vi "Inline CRC-8-CCITT & CRC-8-Maxim.vi"(0 "CRC In":u8 format="%.0x", 1 "CRC-8 Type":T1(ring), 5 "Reset":bool, 7 "Data":u8 format="%.0x", 11 "error in (no error)":errorcluster) -> (4 "CRC":u8 format="%.0x", 15 "error out":errorcluster)   [LabVIEW 2020]
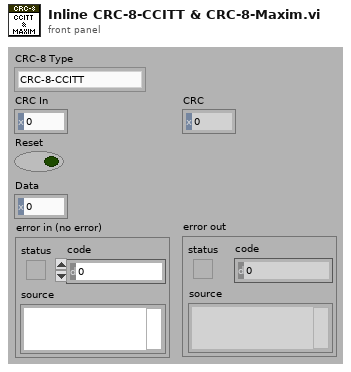
[diagram p1: front panel]
types:
  T1 = enum16{"CRC-8-CCITT", "CRC-8-Maxim 1-Wire (DOW)"}
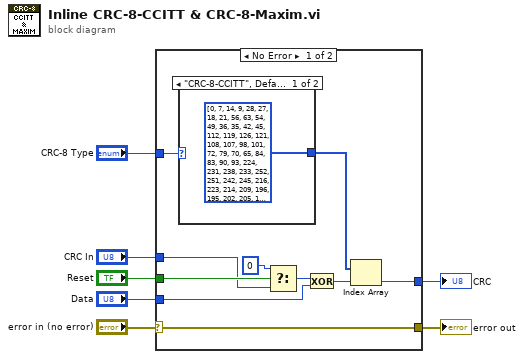
[diagram p0: block diagram]
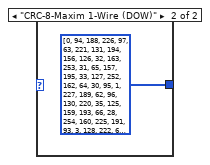
[diagram p2: hidden frame]
diagram:
  n1 = case shown="No Error" "error in (no error)" {
    selector: "error in (no error)" -> [w9 w20]
    tunnel: "Data" -> [w17 _]
    tunnel: "CRC-8 Type" -> [w15 _]
    tunnel: "Reset" -> [w14 _]
    tunnel: [w12 _] -> w4
    tunnel: [w9 w20] -> w2
    tunnel: "CRC In" -> [w8 _]
    frame No Error {
      n2 = case shown="\"CRC-8-CCITT\", Default" w15 {
        tunnel: [u8[] [0, 7, 14, 9, 28, 27, 18, 21, 56, 63, 54, 49, 36, 35, 42, 45, 112, 119, 126, 121, 108, 107, 98, 101, 72, 79, 70, 65, 84, 83, 90, 93, 224, 231, 238, 233, 252, 251, 242, 245, 216, 223, 214, 209, 196, 195, 202, 205, 144, 151, 158, 153, 140, 139, 130, 133, 168, 175, 166, 161, 180, 179, 186, 189, 199, 192, 201, 206, 219, 220, 213, 210, 255, 248, 241, 246, 227, 228, 237, 234, 183, 176, 185, 190, 171, 172, 165, 162, 143, 136, 129, 134, 147, 148, 157, 154, 39, 32, 41, 46, 59, 60, 53, 50, 31, 24, 17, 22, 3, 4, 13, 10, 87, 80, 89, 94, 75, 76, 69, 66, 111, 104, 97, 102, 115, 116, 125, 122, 137, 142, 135, 128, 149, 146, 155, 156, 177, 182, 191, 184, 173, 170, 163, 164, 249, 254, 247, 240, 229, 226, 235, 236, 193, 198, 207, 200, 221, 218, 211, 212, 105, 110, 103, 96, 117, 114, 123, 124, 81, 86, 95, 88, 77, 74, 67, 68, 25, 30, 23, 16, 5, 2, 11, 12, 33, 38, 47, 40, 61, 58, 51, 52, 78, 73, 64, 71, 82, 85, 92, 91, 118, 113, 120, 127, 106, 109, 100, 99, 62, 57, 48, 55, 34, 37, 44, 43, 6, 1, 8, 15, 26, 29, 20, 19, 174, 169, 160, 167, 178, 181, 188, 187, 150, 145, 152, 159, 138, 141, 132, 131, 222, 217, 208, 215, 194, 197, 204, 203, 230, 225, 232, 239, 250, 253, 244, 243] ("first row 2") u8[] [0, 94, 188, 226, 97, 63, 221, 131, 194, 156, 126, 32, 163, 253, 31, 65, 157, 195, 33, 127, 252, 162, 64, 30, 95, 1, 227, 189, 62, 96, 130, 220, 35, 125, 159, 193, 66, 28, 254, 160, 225, 191, 93, 3, 128, 222, 60, 98, 190, 224, 2, 92, 223, 129, 99, 61, 124, 34, 192, 158, 29, 67, 161, 255, 70, 24, 250, 164, 39, 121, 155, 197, 132, 218, 56, 102, 229, 187, 89, 7, 219, 133, 103, 57, 186, 228, 6, 88, 25, 71, 165, 251, 120, 38, 196, 154, 101, 59, 217, 135, 4, 90, 184, 230, 167, 249, 27, 69, 198, 152, 122, 36, 248, 166, 68, 26, 153, 199, 37, 123, 58, 100, 134, 216, 91, 5, 231, 185, 140, 210, 48, 110, 237, 179, 81, 15, 78, 16, 242, 172, 47, 113, 147, 205, 17, 79, 173, 243, 112, 46, 204, 146, 211, 141, 111, 49, 178, 236, 14, 80, 175, 241, 19, 77, 206, 144, 114, 44, 109, 51, 209, 143, 12, 82, 176, 238, 50, 108, 142, 208, 83, 13, 239, 177, 240, 174, 76, 18, 145, 207, 45, 115, 202, 148, 118, 40, 171, 245, 23, 73, 8, 86, 180, 234, 105, 55, 213, 139, 87, 9, 235, 181, 54, 104, 138, 212, 149, 203, 41, 119, 244, 170, 72, 22, 233, 183, 85, 11, 136, 214, 52, 106, 43, 117, 151, 201, 74, 20, 246, 168, 116, 42, 200, 150, 21, 75, 169, 247, 182, 232, 10, 84, 215, 137, 107, 53] ("array")] -> w16
        frame "CRC-8-CCITT", Default {
        }
        frame "CRC-8-Maxim 1-Wire (DOW)" {
        }
      }
      n3 = Select(t=u8 0, s=w14, f=w8) -> (s? t:f=w10:u8)
      n4 = Exclusive Or(1:w17, 2:w10) -> (0:w11:u8)
      n5 = Index Array(array=w16, index=w11) -> (element=w12:u8)
    }
    frame Error {
    }
  }
  "CRC" <- w4
  "error out" <- w2
